vi "TFA Phase Vocoder Online (SubVI).vi"(8 "hop":i32=256, 9 "N":i32=256, 10 "squeeze":dbl=0.5, 11 "STFT coef in":cdb[][](array[numeric])=array513x15[7695 elements]) -> (3 "STFT coef out":cdb[][](array[numeric]))   [LabVIEW 2024]
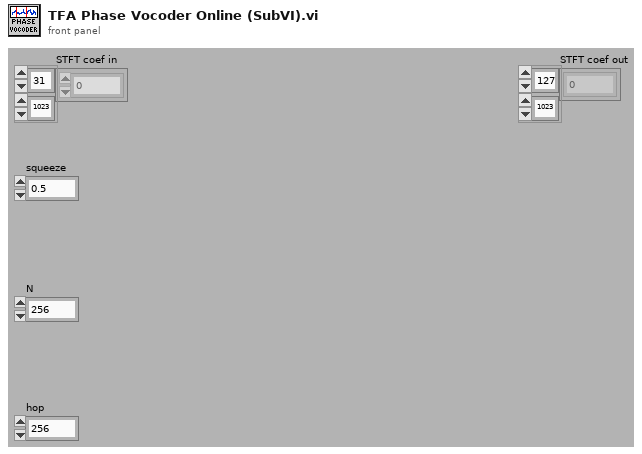
[diagram p1: front panel]
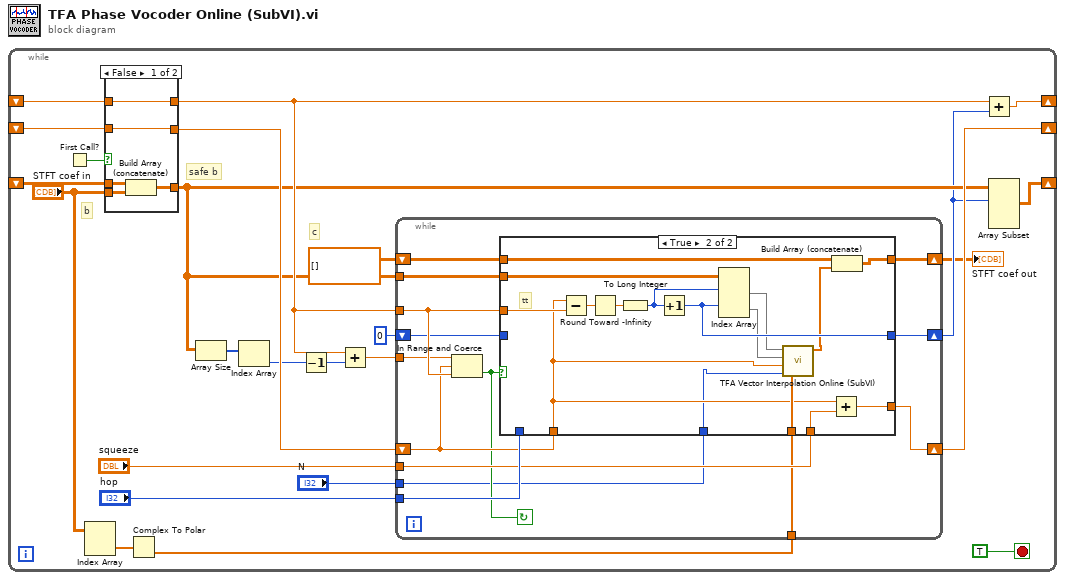
[diagram p0: block diagram]
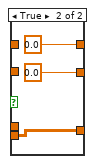
[diagram p3: hidden frame]
diagram:
  n1 = while {
    shift-right: [w19] -> _
    shift-left: _ -> [w20]
    shift-right: [w17] -> _
    shift-left: _ -> [w18]
    shift-right: [w8] -> _
    shift-left: _ -> [w16]
    stop <- TRUE stop-if-true
    # "c"
    # "b"
    # "safe b"
    n2 = First Call?() -> (First Call?: T/F=w22:bool)
    n3 = Index Array(array="STFT coef in") -> (element=w5:cdb[])  [unwired: 2 in]
    n4 = case shown="False" w22 {
      tunnel: [w63 0.0] -> w21
      tunnel: w20 -> [w63 _]
      tunnel: [w62 0.0] -> w14
      tunnel: w18 -> [w62 _]
      tunnel: "STFT coef in" -> [w60 w64]
      tunnel: [w59 w64] -> w9
      tunnel: w16 -> [w61 _]
      frame False {
        n5 = Build Array (concatenate)(w61, w60) -> (w59:cdb[][])
      }
      frame True {
      }
    }
    n6 = Complex To Polar(r * e^(i*theta)=w5) -> (theta=w4:dbl[])  [unwired: 1 out]
    n7 = Array Size(array=w9) -> (size(s)=w13:i32[])
    n8 = Index Array(array=w13) -> (element=w12:i32)  [unwired: 1 in]
    n9 = Decrement(x=w12) -> (x-1=w6:i32)
    n10 = Add(x=w14, y=w6) -> (x+y=w11:dbl)
    n11 = while {
      tunnel: "squeeze" -> [w30]
      shift-right: [w36] -> w2
      shift-left: cdb[][] [] ("initialized array") -> [w37]
      tunnel: "hop" -> [w39]
      shift-right: [w29] -> w19
      shift-left: w21 -> [w34]
      tunnel: w9 -> [w38]
      tunnel: w14 -> [w35]
      tunnel: w11 -> [w33]
      shift-right: [w32] -> w7
      shift-left: 0 -> [w31]
      tunnel: w4 -> [w27]
      tunnel: "N" -> [w26]
      stop <- w28 continue-if-true
      n12 = In Range and Coerce(upper limit=w33, x=w34, lower limit=w35) -> (In Range?=w28:bool)  [unwired: 1 out]
      n13 = case shown="True" w28 {
        tunnel: w39 -> [_ _]
        tunnel: w38 -> [_ w56]
        tunnel: w37 -> [w41 w55]
        tunnel: [w41 w54] -> w36
        tunnel: w35 -> [_ w53]
        tunnel: w34 -> [w40 w45]
        tunnel: [w42 w51] -> w32
        tunnel: w31 -> [w42 _]
        tunnel: w30 -> [_ w50]
        tunnel: [w40 w49] -> w29
        tunnel: w27 -> [_ w48]
        tunnel: w26 -> [_ w44]
        frame False {
        }
        frame True {
          # "tt"
          n14 = Subtract(x=w45, y=w53) -> (x-y=w58:dbl)
          n15 = Round Toward -Infinity(1:w58) -> (0:w57:dbl)
          n16 = To Long Integer(number=w57) -> (32bit integer=w52:i32)
          n17 = Increment(x=w52) -> (x+1=w51:i32)
          n18 = Index Array(array=w56, index (row) #1=w52, index (row) #2=w51) -> (element #1=w47:cdb[], element #2=w46:cdb[])  [unwired: 2 in]
          n19 = call "TFA Vector Interpolation Online (SubVI).vi"("phase 0"=w48, "N"=w44, "new time instance (t)"=w45, "FFT (t1)"=w46, "FFT (t0)"=w47) -> ("interpolation"=w43:cdb[])  [unwired: 1 in, 5 out]
          n20 = Add(x=w45, y=w50) -> (x+y=w49:dbl)
          n21 = Build Array (concatenate)(w55, w43) -> (w54:cdb[][])
        }
      }
    }
    "STFT coef out" <- w2
    n22 = Add(x=w14, y=w7) -> (x+y=w17:dbl)
    n23 = Array Subset(array=w9, index (row)=w7) -> (w8:cdb[][])  [unwired: 3 in]
  }
